vi "GVmotor_init.vi"(8 "err_in":errorcluster, 11 "mWMotor_Port":refnum<visa-resource-name>) -> (0 "error out":errorcluster, 3 "reference out":refnum<visa-resource-name>)   [LabVIEW 2019]
uses:
  <vilib>/Instr/_visa.llb/VISA Flush IO Buffer Mask.ctl
panel:
  in  "Mask":T1=16 items=["Flush Receive Buffer"=16, "Write Transmit Buffer to Device"=32, "Flush Receive Buffer (No I/O)"=64, "Flush Transmit Buffer"=128]
  in  "Message Based Settings:Suppress End Enable":bool
  in  "Message Based Settings:Send End Enable":bool
  in  "Message Based Settings:Termination Character Enable":bool
  in  "Serial Settings:End Mode for Writes":u16(ring)=2 items=["None", "Last Bit", "TermChar", "Break"]
  in  "Serial Settings:End Mode for Reads":u16(ring)=2 items=["None", "Last Bit", "TermChar"]
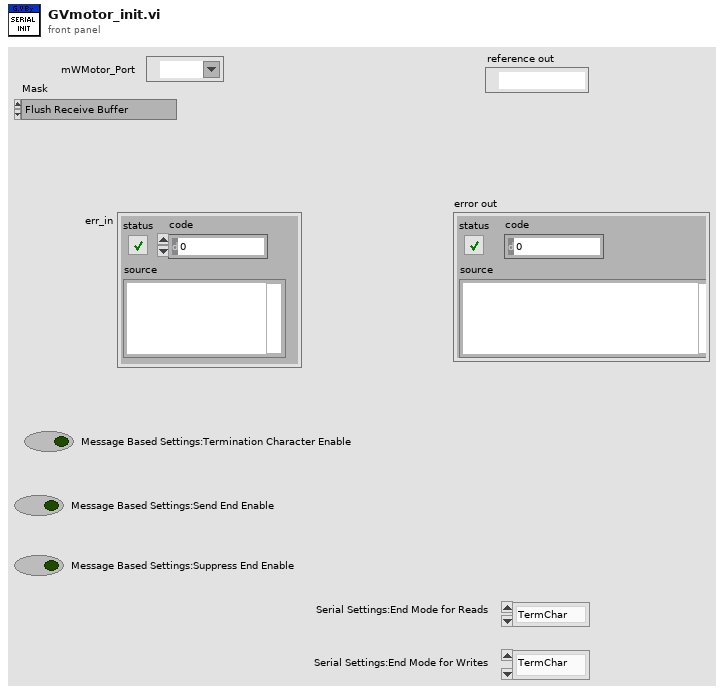
[diagram p1: front panel]
types:
  T1 = typedef "VISA Flush IO Buffer Mask.ctl" = u16
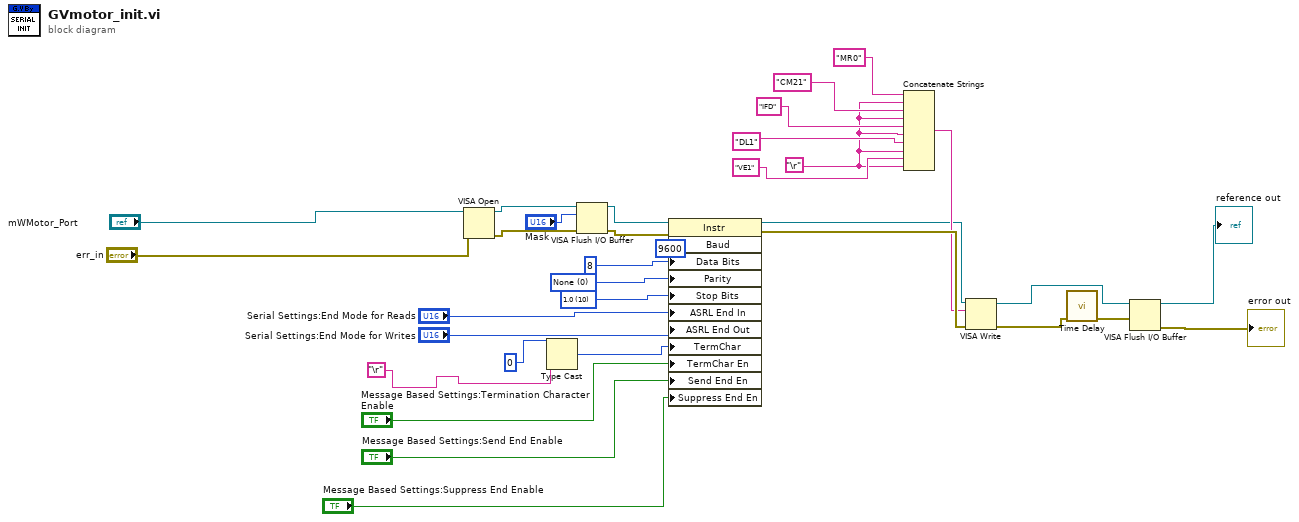
[diagram p0: block diagram]
diagram:
  w1 = "\r"
  w30 = u16 10 items=["1.0"=10, "1.5"=15, "2.0"=20] ("Serial Settings:Stop Bits")
  w31 = u16 0 items=["None", "Odd", "Even", "Mark", "Space"] ("Serial Settings:Parity")
  n1 = VISA Open(error in (no error)="err_in", VISA resource name="mWMotor_Port") -> (VISA resource name=w20:refnum<visa-resource-name>, error out=w17:errorcluster)  [unwired: 3 in]
  n2 = Type Cast(type=u8 0, x="\r") -> (*(type *) &x=w26:u8)
  n3 = VISA Flush I/O Buffer(VISA resource name=w20, mask (16)="Mask", error in (no error)=w17) -> (VISA resource name out=w19:refnum<visa-resource-name>, error out=w18:errorcluster)
  n4 = property class="Instr"(reference=w19, error in=w18, "Baud"=u32 9600 ("Serial Settings:Baud Rate"), "Data Bits"=u16 8 ("Serial Settings:Data Bits"), "Parity"=w31, "Stop Bits"=w30, "ASRL End In"="Serial Settings:End Mode for Reads", "ASRL End Out"="Serial Settings:End Mode for Writes", "TermChar"=w26, "TermChar En"="Message Based Settings:Termination Character Enable", "Send End En"="Message Based Settings:Send End Enable", "Suppress End En"="Message Based Settings:Suppress End Enable") -> (reference out=w12:refnum<visa-resource-name>, error out=w15:errorcluster)
  n5 = Concatenate Strings("MR0" ("string"), w1, "CM21" ("string"), w1, "IFD" ("string"), w1, "DL1" ("string"), w1, "VE1" ("string"), w1) -> (w13:string)
  n6 = VISA Write(VISA resource name=w12, write buffer=w13, error in (no error)=w15) -> (VISA resource name out=w7:refnum<visa-resource-name>, error out=w11:errorcluster)  [unwired: 1 out]
  n7 = call "Time Delay"("error in (no error)"=w11) -> ("error out"=w10:errorcluster)  [unwired: 10 in]
  n8 = VISA Flush I/O Buffer(VISA resource name=w7, error in (no error)=w10) -> (VISA resource name out=→"reference out":refnum<visa-resource-name>, error out=→"error out":errorcluster)  [unwired: 1 in]
